vi "numeric operations 2.vi"() -> ()   [LabVIEW 2020]
panel:
  out "quotient":dbl
  out "remainder":dbl
  in  "input 2":dbl
  in  "input 1":dbl
  out "reciprocal":dbl
  in  "input":dbl
  out "negative":dbl
  in  "input":dbl
  out "square root":dbl
  out "square":dbl
  in  "input":dbl
  # "Numeric operation"
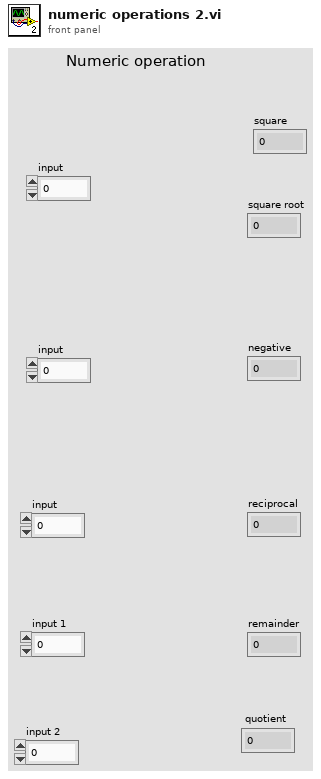
[diagram p1: front panel]
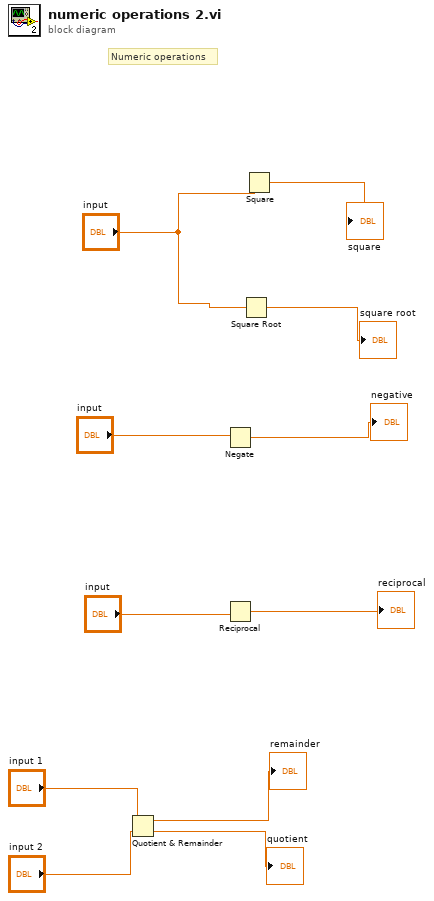
[diagram p0: block diagram]
diagram:
  # "Numeric operations"
  n1 = Quotient & Remainder(x="input 1", y="input 2") -> (x-y*floor(x/y)=→"remainder":dbl, floor(x/y)=→"quotient":dbl)
  n2 = Negate(x="input") -> (-x=→"negative":dbl)
  n3 = Reciprocal(x="input") -> (1/x=→"reciprocal":dbl)
  n4 = Square Root(x="input") -> (sqrt(x)=→"square root":dbl)
  n5 = Square(x="input") -> (x^2=→"square":dbl)
